vi "ep_Check Waveform Continuity.vi"(6 "initial conditions":T1, 7 "reset? (F)":bool, 8 "error in (no error)":errorcluster, 11 "signal":waveform(dbl)) -> (0 "error out":errorcluster, 4 "final conditions":T1)   [LabVIEW 2014, in "NI_EP_Motor Monitoring.lvlib"]
uses:
  <vilib>/addons/Electrical Power/Motor Monitoring/NI_EP_Motor Monitoring.lvlib
  <vilib>/addons/Electrical Power/Motor Monitoring/subVIs/ep_Initial Conditions for Air Gap.ctl
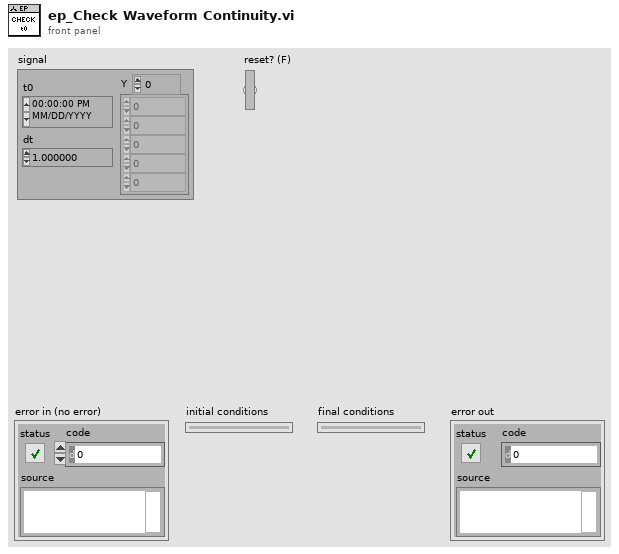
[diagram p1: front panel]
types:
  T1 = typedef "NI_EP_Motor Monitoring.lvlib/ep_Initial Conditions for Air Gap.ctl" = cluster{"integration state in A":cluster{"initial value":dbl, "initial integration":dbl}, "integration state in B":cluster{"initial value":dbl, "initial integration":dbl}, "integrated state A":dbl[], "integrated state B":dbl[], "previous length":i32, "loss and polepair":cluster{"Pstray [W]":dbl, "Pfric [W]":dbl, "Polepair #":i32, "synchronous speed [RPM]":dbl}, "expected timestamp":timestamp}
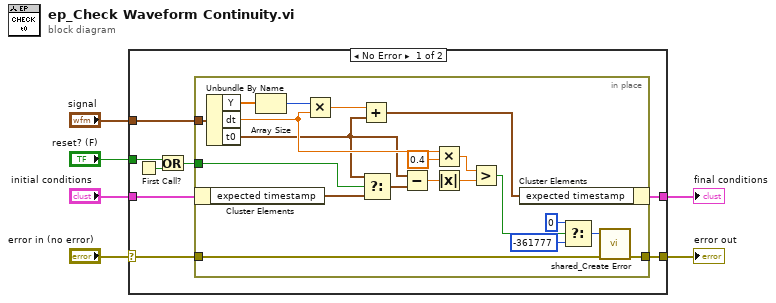
[diagram p0: block diagram]
diagram:
  n1 = case shown="No Error" "error in (no error)" {
    selector: "error in (no error)" -> [w14 w35]
    tunnel: [w7 w35] -> w5
    tunnel: "initial conditions" -> [w13 _]
    tunnel: "signal" -> [w12 _]
    tunnel: "reset? (F)" -> [w9 _]
    tunnel: [w8 _] -> w1
    frame No Error {
      n2 = First Call?() -> (First Call?: T/F=w10:bool)
      n3 = Or(x=w9, y=w10) -> (x .or. y?=w11:bool)
      n4 = in-place {
        in-place-border: w14 -> [w18]
        in-place-border: w12 -> [w34]
        in-place-border: w11 -> [w30]
        in-place-border: [w17] -> w7
        n5 = in-place-cluster #1(w13) -> ("expected timestamp"=w29:timestamp)
        n6 = Unbundle By Name(w34) -> ("Y"=w33:dbl[], "dt"=w26:dbl, "t0"=w15:timestamp)
        n7 = Array Size(array=w33) -> (size(s)=w32:i32)
        n8 = Multiply(x=w32, y=w26) -> (x*y=w31:dbl)
        n9 = Add(x=w31, y=w15) -> (x+y=w22:timestamp)
        n10 = Select(t=w15, s=w30, f=w29) -> (s? t:f=w28:timestamp)
        n11 = Subtract(x=w15, y=w28) -> (x-y=w27:dbl)
        n12 = Multiply(x=w26, y=0.4) -> (x*y=w23:dbl)
        n13 = Absolute Value(x=w27) -> (abs(x)=w24:dbl)
        n14 = Greater?(x=w23, y=w24) -> (0:w16:bool)
        n15 = in-place-cluster #1("expected timestamp"=w22) -> (w8:T1)
        n16 = Select(t=0, s=w16, f=-361777 ("error code (0)")) -> (s? t:f=w19:i32)
        n17 = call <vilib>:"shared_Create Error.vi"("error in (no error)"=w18, "error code (0)"=w19) -> ("error out"=w17:errorcluster)  [unwired: 9 in]
      }
    }
    frame Error {
    }
  }
  "error out" <- w5
  "final conditions" <- w1
